vi "Cooldown resistor monitor.vi"() -> ()   [LabVIEW 2010]
uses:
  <instrlib>/Keithley 2000/Public/Configure/Configure 2 Wire Resistance.vi
  <vilib>/Utility/file.llb/Write To Spreadsheet File (string).vi
  <instrlib>/Keithley 2000/Keithley 2000.lvlib
panel:
  out "channel names":string[](array[string])
  out "latest values":dbl[](array[numeric])
  in  "samples per second":u32=1
  out "error out":errorcluster
  out "XY Graph":cluster{timestamp[], dbl[]}[](graph)
  in  "stop":bool
  in  "stop channel":i32=8
  in  "start channel":i32=1
  in  "error in (no error)":errorcluster
  in  "VISA resource name":refnum<visa-resource-name>="GPIB::16"
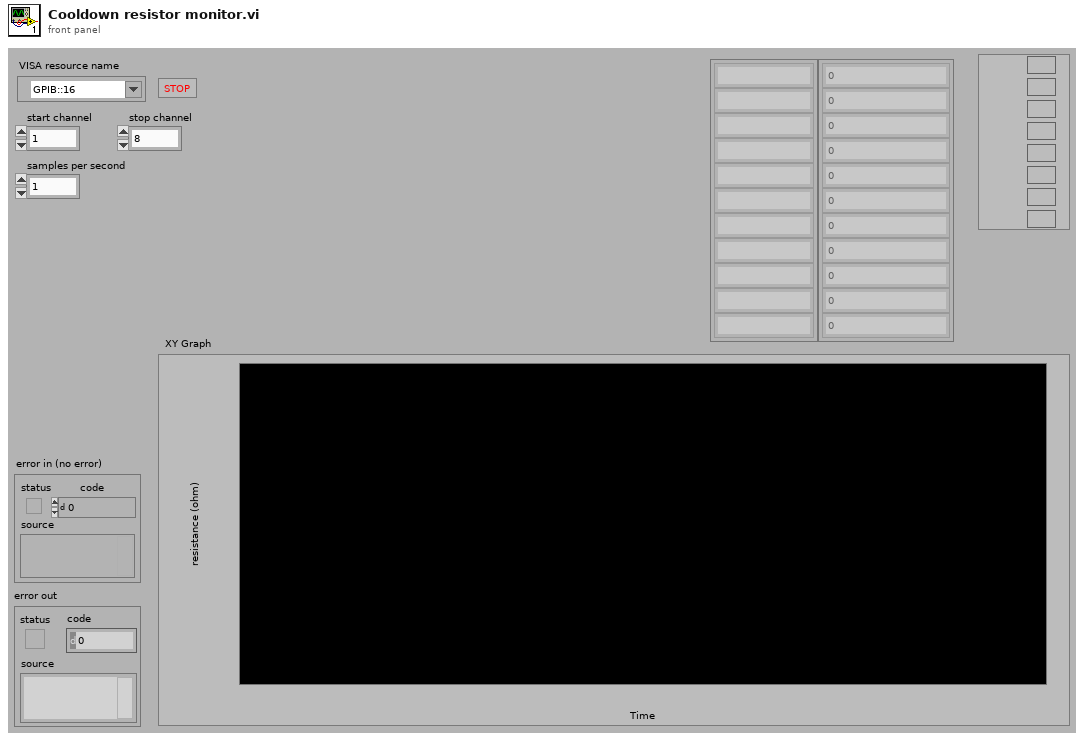
[diagram p1: front panel]
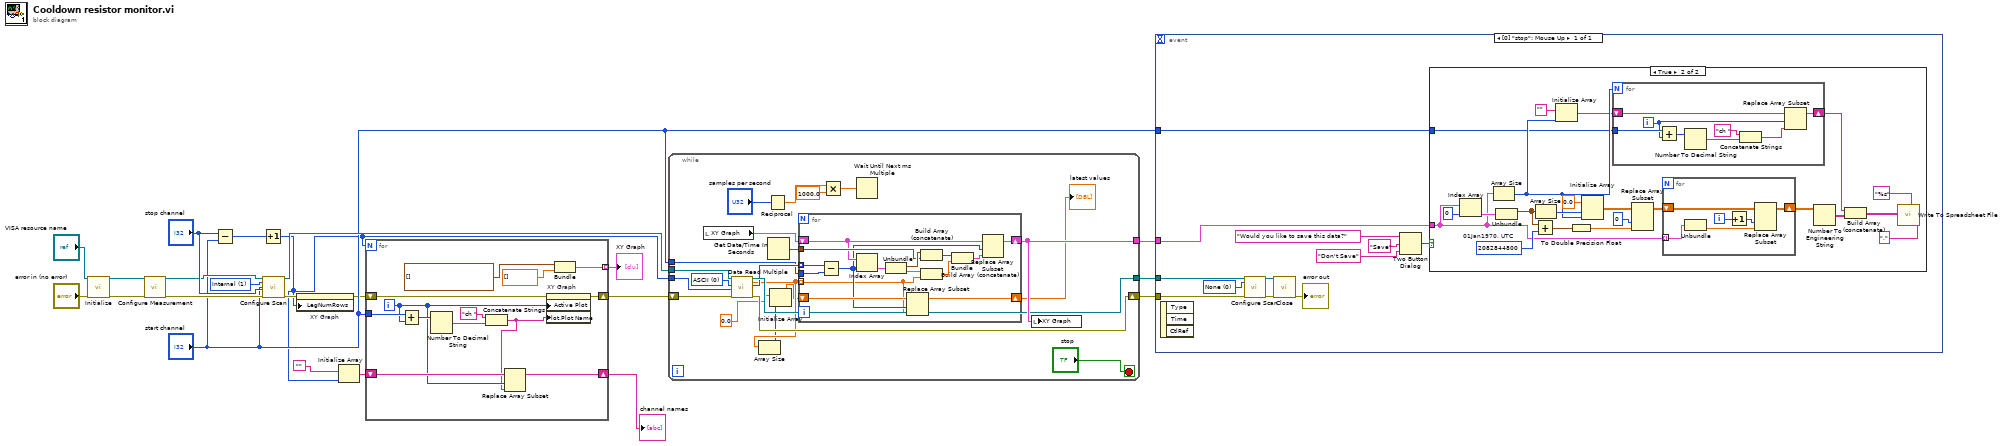
[diagram p0: block diagram]
diagram:
  w20 = u16 1 items=["None", "Internal", "External"] ("Scan Mode (0: None)")
  n1 = call <instrlib>:"Initialize.vi"("VISA resource name"="VISA resource name", "error in (no error)"="error in (no error)") -> ("VISA resource name out"=w11:refnum<visa-resource-name>, "error out"=w10:errorcluster)  [unwired: 16 in]
  n2 = call-poly <instrlib>:"Configure Measurement.vi"("VISA resource name"=w11, "error in (no error)"=w10) -> ("VISA resource name out"=w8:refnum<visa-resource-name>, "error out"=w9:errorcluster)  [unwired: 16 in]
  n3 = Subtract(x="stop channel", y="start channel") -> (x-y=w17:i32)
  n4 = Increment(x=w17) -> (x+1=w3:i32)
  n5 = call <instrlib>:"Configure Scan.vi"("VISA resource name"=w8, "Scan Mode (0: None)"=w20, "Starting Channel (1)"="start channel", "Stopping Channel (10)"="stop channel", "error in (no error)"=w9) -> ("VISA resource name out"=w19:refnum<visa-resource-name>, "error out"=w6:errorcluster)  [unwired: 13 in]
  n6 = property on="XY Graph" class="XYGraph (strict)"(error in=w6, "LegNumRows"=w3) -> (error out=w5:errorcluster)  [unwired: 1 in, 1 out]
  n7 = Initialize Array("", w3) -> (w2:string[])
  n8 = for {
    N: w3 -> [_]
    shift-right: [w34] -> w16
    shift-left: w5 -> [w35]
    tunnel: "start channel" -> [w32]
    tunnel: [w27] -> w15 mode=indexing
    shift-right: [w23] -> w1
    shift-left: w2 -> [w26]
    i -> [w25]
    n9 = Add(x=w32, y=w25) -> (x+y=w31:i32)
    n10 = Number To Decimal String(number=w31) -> (decimal integer string=w30:string)  [unwired: 1 in]
    n11 = Concatenate Strings("ch " ("string"), w30) -> (w24:string)
    n12 = Replace Array Subset(array=w26, new element=w24, index=w25) -> (w23:string[])
    n13 = property on="XY Graph" class="XYGraph (strict)"(error in=w35, "Active Plot"=w25, "Plot.Plot Name"=w24) -> (error out=w34:errorcluster)  [unwired: 1 in, 1 out]
    n14 = Bundle(timestamp[] [], dbl[] []) -> (w27:cluster{timestamp[], dbl[]})  [unwired: 1 in]
  }
  "XY Graph" <- w15
  "channel names" <- w1
  n15 = while {
    tunnel: w19 -> [w55]
    tunnel: w3 -> [w53]
    tunnel: [w50] -> w14
    tunnel: [w49] -> w13
    shift-right: [w48] -> w12
    shift-left: w16 -> [w54]
    tunnel: "start channel" -> [w43]
    stop <- "stop" stop-if-true
    w45 = u16 0 items=["ASCII", "Single Precision", "Double Precision"] ("Format (0: ASCII)")
    n16 = local read "XY Graph"() -> (w52:cluster{timestamp[], dbl[]}[])
    n17 = call <instrlib>:"Data Read Multiple.vi"("VISA resource name"=w55, "Format (0: ASCII)"=w45, "Number of Readings (100)"=w53, "error in (no error)"=w54) -> ("VISA resource name out"=w49:refnum<visa-resource-name>, "Data"=w39:dbl[], "Channels"=w44:i32[], "error out"=w48:errorcluster)  [unwired: 11 in, 1 out]
    n18 = Array Size(array=w39) -> (size(s)=w38:i32)
    n19 = Reciprocal(x="samples per second") -> (1/x=w46:dbl)
    n20 = Get Date/Time In Seconds() -> (seconds since 1Jan1904=w51:timestamp)
    n21 = Initialize Array(0.0, w38) -> (w37:dbl[])
    n22 = for {
      tunnel: w51 -> [w70]
      tunnel: w39 -> [w58] mode=indexing
      tunnel: w44 -> [w66] mode=indexing
      tunnel: w43 -> [w65]
      shift-right: [w61] -> w50
      shift-left: w52 -> [w63]
      shift-right: [w57] -> w36
      shift-left: w37 -> [w60]
      n23 = Subtract(x=w66, y=w65) -> (x-y=w59:i32)
      n24 = Index Array(array=w63, index=w59) -> (element=w64:cluster{timestamp[], dbl[]})
      n25 = Unbundle(w64) -> (w71:timestamp[], w69:dbl[])
      n26 = Replace Array Subset(array=w60, new element=w58, index=w59) -> (w57:dbl[])
      n27 = Build Array (concatenate)(w71, w70) -> (w67:timestamp[])
      n28 = Build Array (concatenate)(w69, w58) -> (w68:dbl[])
      n29 = Bundle(w67, w68) -> (w62:cluster{timestamp[], dbl[]})  [unwired: 1 in]
      n30 = Replace Array Subset(array=w63, new element=w62, index=w59) -> (w61:cluster{timestamp[], dbl[]}[])
    }
    "latest values" <- w36
    n31 = Multiply(x=w46, y=1000.0) -> (x*y=w42:dbl)
    n32 = Wait Until Next ms Multiple(millisecond multiple=w42) -> ()  [unwired: 1 out]
    n33 = local write "XY Graph"(w50) -> ()
  }
  n34 = event shown="[0] \"stop\": Mouse Up" {
    selector: _ -> [_]
    dyn-events: _ -> [_]
    timeout: _ -> [_]
    tunnel: w14 -> [w79]
    tunnel: "start channel" -> [w78]
    tunnel: w13 -> [w75]
    tunnel: w12 -> [w76]
    event "stop": Mouse Up {
      w72 = u16 0 items=["None", "Internal", "External"] ("Scan Mode (0: None)")
      n35 = event-data() -> ()  [unwired: 1 in, 3 out]
      n36 = call <instrlib>:"Configure Scan.vi"("VISA resource name"=w75, "Scan Mode (0: None)"=w72, "error in (no error)"=w76) -> ("VISA resource name out"=w74:refnum<visa-resource-name>, "error out"=w73:errorcluster)  [unwired: 15 in]
      n37 = call <instrlib>:"Close.vi"("VISA resource name"=w74, "error in (no error)"=w73) -> ("error out"=→"error out":errorcluster)  [unwired: 17 in]
      n38 = Two Button Dialog(message="Would you like to save this data?", 1:"Don't Save" ("F button name (\"Cancel\")"), 2:"Save" ("T button name (\"OK\")")) -> (T button?=w80:bool)
      n39 = case shown="True" w80 {
        tunnel: w79 -> [_ w94]
        tunnel: w78 -> [_ w90]
        frame False {
        }
        frame True {
          w103 = u64 2082844800  # 01Jan1970, UTC
          n40 = Index Array(array=w94, index=0) -> (element=w104:cluster{timestamp[], dbl[]})
          n41 = Array Size(array=w94) -> (size(s)=w92:i32)
          n42 = Unbundle(w104) -> (w102:timestamp[])  [unwired: 1 out]
          n43 = Add(x=w102, y=w103) -> (x+y=w98:timestamp[])
          n44 = Array Size(array=w102) -> (size(s)=w96:i32)
          n45 = Initialize Array("", w92) -> (w91:string[])
          n46 = To Double Precision Float(number=w98) -> (double precision float=w97:dbl[])
          n47 = Initialize Array(0.0, w96, w92) -> (w101:dbl[][])
          n48 = for {
            N: w92 -> [_]
            shift-right: [w106] -> w89
            shift-left: w91 -> [w113]
            tunnel: w90 -> [w110]
            i -> [w109]
            n49 = Add(x=w110, y=w109) -> (x+y=w108:i32)
            n50 = Number To Decimal String(number=w108) -> (decimal integer string=w107:string)  [unwired: 1 in]
            n51 = Concatenate Strings("ch " ("string"), w107) -> (w112:string)
            n52 = Replace Array Subset(array=w113, new element=w112, index=w109) -> (w106:string[])
          }
          n53 = Replace Array Subset(array=w101, new element=w97, index (col)=0 ("disabled index (col)")) -> (w95:dbl[][])  [unwired: 1 in]
          n54 = for {
            shift-right: [w114] -> w88
            shift-left: w95 -> [w115]
            tunnel: w94 -> [w119] mode=indexing
            i -> [w118]
            n55 = Unbundle(w119) -> (w116:dbl[])  [unwired: 1 out]
            n56 = Increment(x=w118) -> (x+1=w117:i32)
            n57 = Replace Array Subset(array=w115, new element=w116, index (col)=w117) -> (w114:dbl[][])  [unwired: 1 in]
          }
          n58 = Number To Engineering String(4:w88) -> (0:w87:string[][])  [unwired: 3 in]
          n59 = Build Array (concatenate)(w89, w87) -> (w84:string[][])
          n60 = call-poly <vilib>:"Write To Spreadsheet File.vi"("delimiter (\\t)"="," ("delimiter (\\t)"), "format (%s)"="%s" ("format (%.3f)"), "2D data"=w84) -> ()  [unwired: 5 in, 1 out]
        }
      }
    }
  }
